vi "Benchmark Running.vi"(8 "error in (no error)":errorcluster, 11 "CIFCorePlugin in":refnum<class "CIFCorePlugin.lvclass">) -> (0 "error out":errorcluster, 3 "CIFCorePlugin out":refnum<class "CIFCorePlugin.lvclass">)   [LabVIEW 2021, in "CIFCorePlugin.lvclass"]
uses:
  CIFCorePlugin.lvclass
  CIFCoreCommon/CIFCoreCommon.lvlib
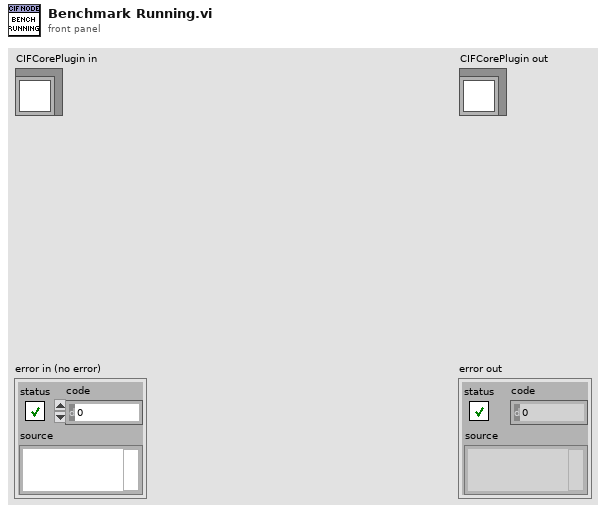
[diagram p1: front panel]
types:
  T1 = typedef "CIFCoreCommon.lvlib/Timing Stats Base.ctl" = cluster{"Max":i32, "Min":i32}
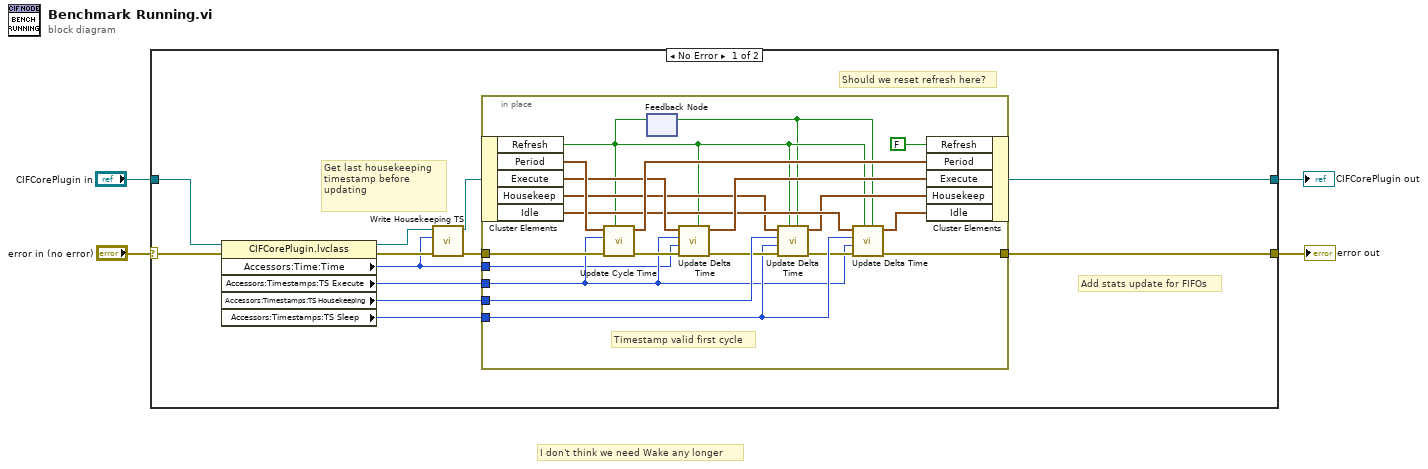
[diagram p0: block diagram]
diagram:
  # "I don't think we need Wake any longer"
  n1 = case shown="No Error" "error in (no error)" {
    selector: "error in (no error)" -> [w15 w38]
    tunnel: [w5 w38] -> w1
    tunnel: [w6 w37] -> w2
    tunnel: "CIFCorePlugin in" -> [w16 w37]
    frame No Error {
      # "Get last housekeeping timestamp before updating"
      # "Should we reset refresh here?"
      # "Add stats update for FIFOs"
      n2 = property class="CIFCorePlugin.lvclass"(reference=w16, error in=w15) -> (reference out=w9:refnum<class "CIFCorePlugin.lvclass">, error out=w11:errorcluster, "Accessors:Time:Time"=w7:u64, "Accessors:Timestamps:TS Execute"=w12:u64, "Accessors:Timestamps:TS Housekeeping"=w13:u64, "Accessors:Timestamps:TS Sleep"=w14:u64)
      n3 = call "Write Housekeeping TS.vi"("error in (no error)"=w11, "Housekeeping"=w7, "CIFCorePlugin in"=w9) -> ("error out"=w10:errorcluster, "CIFCorePlugin out"=w8:refnum<class "CIFCorePlugin.lvclass">)  [unwired: 7 in]
      n4 = in-place {
        in-place-border: w12 -> [w20]
        in-place-border: w13 -> [w29]
        in-place-border: w14 -> [w27]
        in-place-border: w10 -> [w33]
        in-place-border: [w26] -> w5
        in-place-border: w7 -> [w19]
        # "Timestamp valid first cycle"
        n5 = in-place-cluster #1(w8) -> ("Refresh"=w18:bool, "Period"=w36:T1, "Execute"=w31:T1, "Housekeep"=w24:T1, "Idle"=w25:T1)
        n6 = call "Update Cycle Time.vi"("Initialize"=w18, "error in (no error)"=w33, "T1"=w20, "Timing in"=w36) -> ("error out"=w32:errorcluster, "Timing out"=w34:cluster{"Max":i32, "Min":i32})  [unwired: 6 in]
        n7 = feedback-in #2(w18) -> ()
        n8 = feedback #2() -> (w17:bool)  [unwired: 1 in]
        n9 = call "Update Delta Time.vi"("reinit"=w18, "error in (no error)"=w32, "T2"=w19, "T1"=w20, "Timing in"=w31) -> ("error out"=w28:errorcluster, "Timing out"=w30:cluster{"Max":i32, "Min":i32})  [unwired: 5 in]
        n10 = call "Update Delta Time.vi"("reinit"=w17, "skip"=w18, "error in (no error)"=w28, "T2"=w27, "T1"=w29, "Timing in"=w24) -> ("error out"=w21:errorcluster, "Timing out"=w22:cluster{"Max":i32, "Min":i32})  [unwired: 4 in]
        n11 = call "Update Delta Time.vi"("reinit"=w17, "skip"=w18, "error in (no error)"=w21, "T2"=w20, "T1"=w27, "Timing in"=w25) -> ("error out"=w26:errorcluster, "Timing out"=w23:cluster{"Max":i32, "Min":i32})  [unwired: 4 in]
        n12 = in-place-cluster #1("Refresh"=FALSE, "Period"=w34, "Execute"=w30, "Housekeep"=w22, "Idle"=w23) -> (w6:refnum<class "CIFCorePlugin.lvclass">)
      }
    }
    frame Error {
    }
  }
  "error out" <- w1
  "CIFCorePlugin out" <- w2
